vi "Example Countdown Timer.vi"(11 "Start Logging":bool) -> (3 "Valid for Logging":bool)   [LabVIEW 2018]
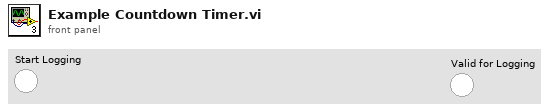
[diagram p1: front panel]
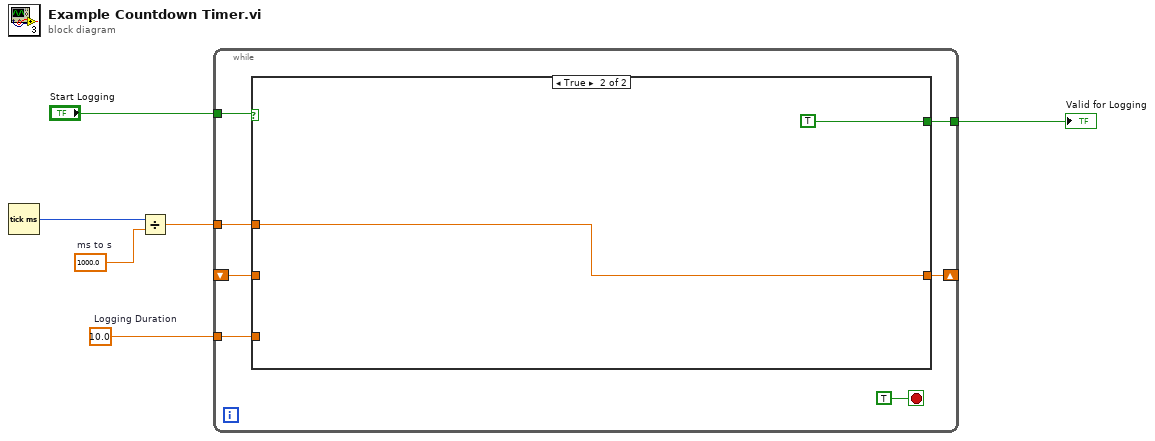
[diagram p0: block diagram]
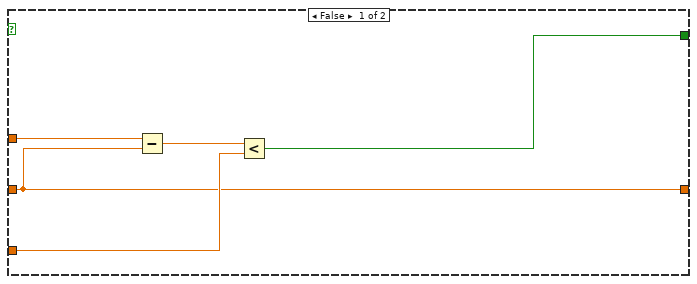
[diagram p2: hidden frame]
diagram:
  w3 = 1000.0  # ms to s
  w5 = 10.0  # Logging Duration
  n1 = Tick Count (ms)() -> (millisecond timer value=w4:u32)
  n2 = Divide(x=w4, y=w3) -> (x/y=w2:dbl)
  n3 = while {
    tunnel: "Start Logging" -> [w13]
    tunnel: w5 -> [w12]
    tunnel: w2 -> [w11]
    shift-right: [w10] -> _
    shift-left: _ -> [w9]
    tunnel: [w7] -> w1
    stop <- TRUE stop-if-true
    n4 = case shown="True" w13 {
      tunnel: w12 -> [w16 _]
      tunnel: w11 -> [w18 w19]
      tunnel: [w15 w19] -> w10
      tunnel: w9 -> [w15 _]
      tunnel: [w14 TRUE] -> w7
      frame False {
        n5 = Subtract(x=w18, y=w15) -> (x-y=w17:dbl)
        n6 = Less?(x=w17, y=w16) -> (x < y?=w14:bool)
      }
      frame True {
      }
    }
  }
  "Valid for Logging" <- w1
